vi "struct_abs_con_X_pT.vi"(0 "Reference working pair (Input)":i64, 5 "Pressure in Pa (Input)":dbl, 7 "Temperature in K (Input)":dbl, 11 "Error (Input)":errorcluster) -> (4 "Concentration in kg/kg (Output)":dbl, 15 "Error (Output)":errorcluster)   [LabVIEW 2017]
doc: "abs_con_X_pT:\n * -------------\n *\n * Calculates equilibrium concentration X in kg/kg depending on equilibrium\n * pressure p in Pa and equilibrium temperature T in K.\n *\n * Parameters:\n * -----------\n * double p_Pa:\n * Equilibrium pressure in Pa.\n * double T_K:\n * Equilibrium temperature in K.\n * struct *WorkingPair:\n * Pointer of WorkingPair-struct.\n *\n * Returns:\n * --------\n * double:\n * Equilibrium concentration in kg/kg.\n *\n * Remarks:\n * --------\n * This function is only valid for isotherm models based on the conventional\n * approach.\n *\n * History: \n * --------\n * 07/14/2021, by Jannik Driesel (supervised by Mirko Engelpracht):\n * First implementation."
uses:
  data/win32bit/libsorpPropLib.dll
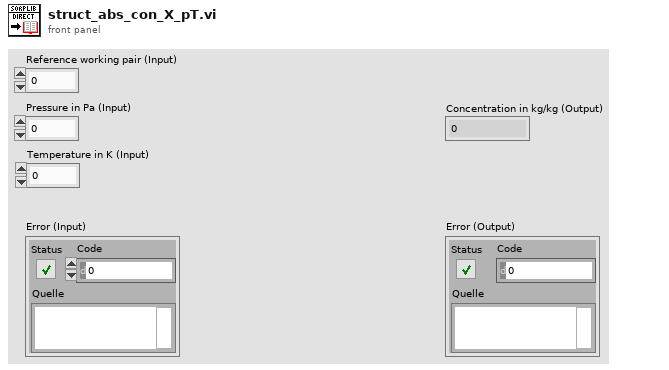
[diagram p1: front panel]
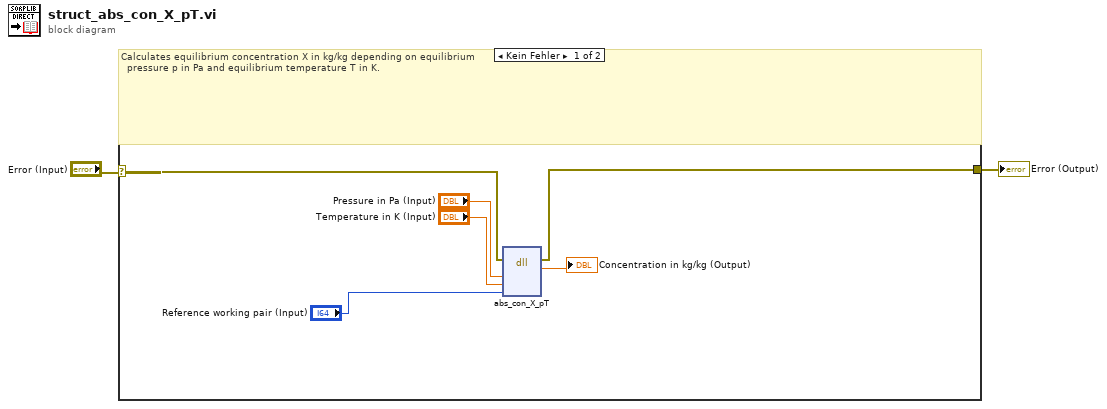
[diagram p0: block diagram]
diagram:
  n1 = case shown="Kein Fehler" "Error (Input)" {
    selector: "Error (Input)" -> [w8 w9]
    tunnel: [w7 w9] -> w2
    frame No Error {
      # "Calculates equilibrium concentration X in kg/kg depending on equilibrium\n  pressure p in Pa and equilibrium temperature T in K."
      n2 = dll-call lib="D:/Driesel/SorpLibLocal/LabVIEW_wrapper/data/win32bit/libsorpPropLib.dll" fn="abs_con_X_pT"(error in=w8, "p_Pa"="Pressure in Pa (Input)", "T_K"="Temperature in K (Input)", "workingPair"="Reference working pair (Input)") -> (error out=w7:errorcluster, "X_kgkg"=→"Concentration in kg/kg (Output)":dbl)  [unwired: 5 in, 1 out]
    }
    frame Error {
      # "Error - No calculations"
    }
  }
  "Error (Output)" <- w2
